vi "Setup array.vi"() -> (3 "output array":string[](array[string]))   [LabVIEW 2014]
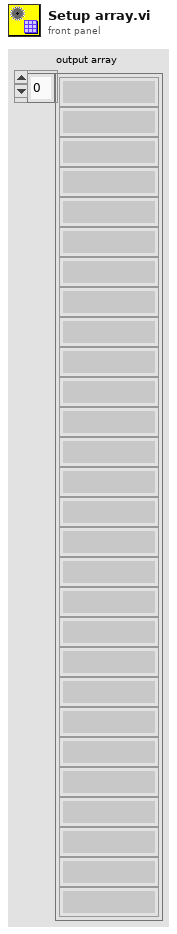
[diagram p1: front panel]
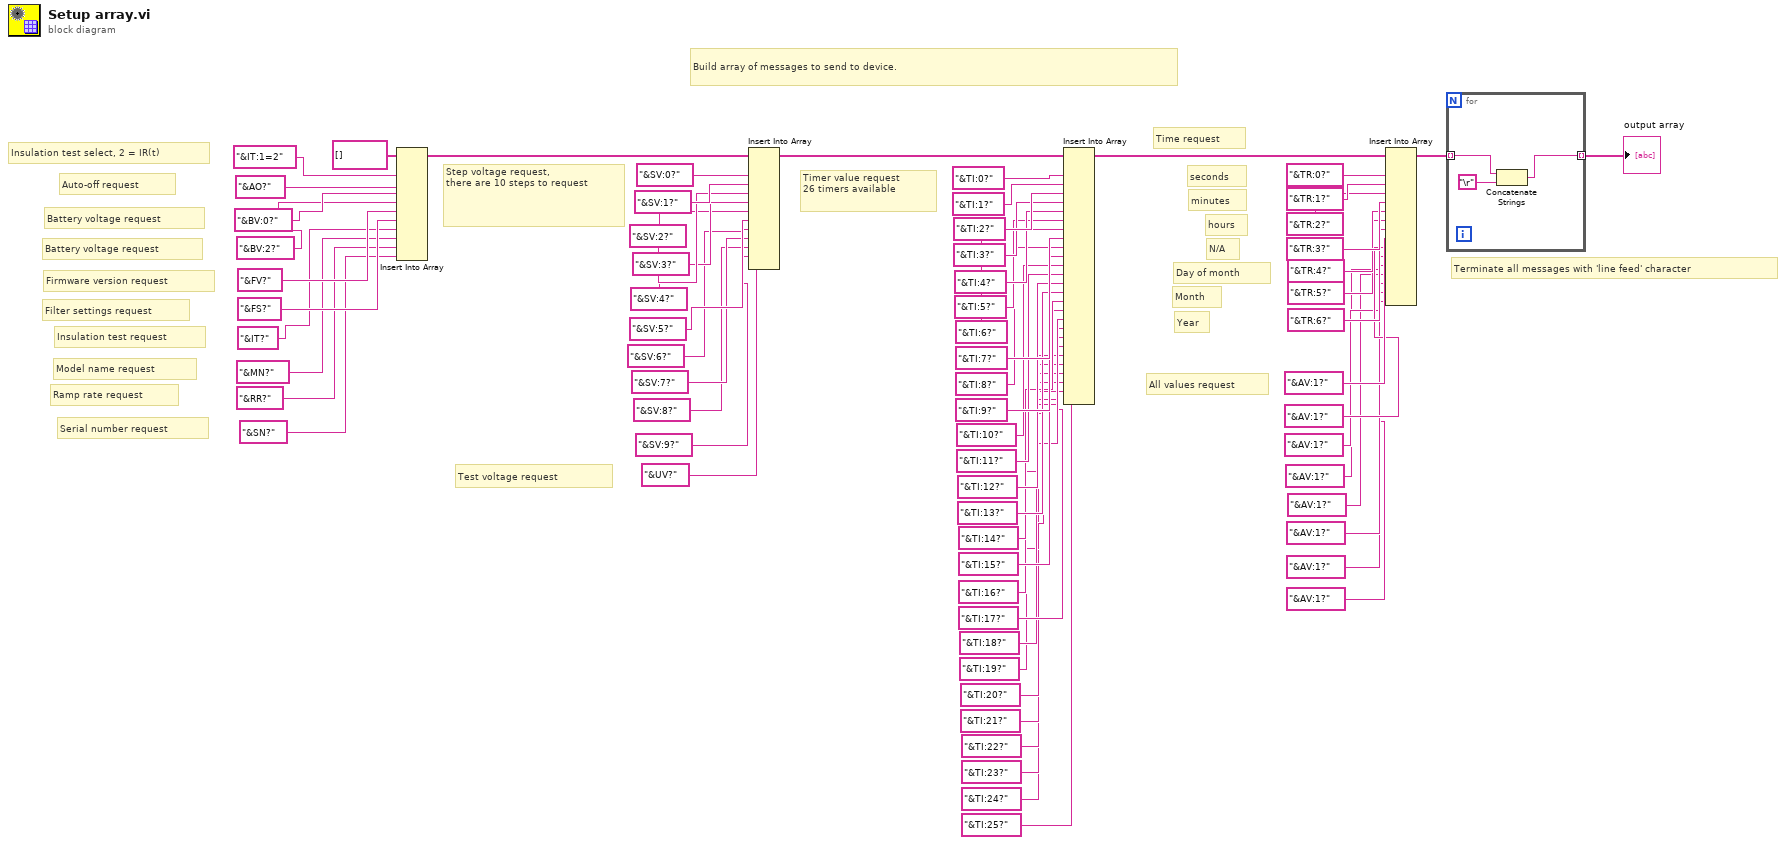
[diagram p0: block diagram]
diagram:
  # "Terminate all messages with 'line feed' character"
  # "All values request"
  # "Year"
  # "Month"
  # "Day of month"
  # "N/A"
  # "hours"
  # "minutes"
  # "seconds"
  # "Time request"
  # "Timer value request\n26 timers available"
  # "Test voltage request"
  # "Step voltage request,\nthere are 10 steps to request"
  # "Build array of messages to send to device."
  # "Serial number request"
  # "Ramp rate request"
  # "Model name request"
  # "Insulation test request"
  # "Filter settings request"
  # "Firmware version request"
  # "Battery voltage request"
  # "Battery voltage request"
  # "Auto-off request"
  # "Insulation test select, 2 = IR(t)"
  n1 = Insert Into Array(array=string[] [], new element #1="&IT:1=2", new element #2="&AO?", new element #3="&BV:0?", new element #4="&BV:2?", new element #5="&FV?", new element #6="&FS?", new element #7="&IT?", new element #8="&MN?", new element #9="&RR?", new element #10="&SN?") -> (w55:string[])  [unwired: 1 in]
  n2 = Insert Into Array(array=w55, new element #1="&SV:0?", new element #2="&SV:1?", new element #3="&SV:2?", new element #4="&SV:3?", new element #5="&SV:4?", new element #6="&SV:5?", new element #7="&SV:6?", new element #8="&SV:7?", new element #9="&SV:8?", new element #10="&SV:9?", new element #11="&UV?") -> (w19:string[])  [unwired: 1 in]
  n3 = Insert Into Array(array=w19, new element #1="&TI:0?", new element #2="&TI:1?", new element #3="&TI:2?", new element #4="&TI:3?", new element #5="&TI:4?", new element #6="&TI:5?", new element #7="&TI:6?", new element #8="&TI:7?", new element #9="&TI:8?", new element #10="&TI:9?", new element #11="&TI:10?", new element #12="&TI:11?", new element #13="&TI:12?", new element #14="&TI:13?", new element #15="&TI:14?", new element #16="&TI:15?", new element #17="&TI:16?", new element #18="&TI:17?", new element #19="&TI:18?", new element #20="&TI:19?", new element #21="&TI:20?", new element #22="&TI:21?", new element #23="&TI:22?", new element #24="&TI:23?", new element #25="&TI:24?", new element #26="&TI:25?") -> (w11:string[])  [unwired: 1 in]
  n4 = Insert Into Array(array=w11, new element #1="&TR:0?", new element #2="&TR:1?", new element #3="&TR:2?", new element #4="&TR:3?", new element #5="&TR:4?", new element #6="&TR:5?", new element #7="&TR:6?", new element #8="&AV:1?", new element #9="&AV:1?", new element #10="&AV:1?", new element #11="&AV:1?", new element #12="&AV:1?", new element #13="&AV:1?", new element #14="&AV:1?", new element #15="&AV:1?") -> (w10:string[])  [unwired: 1 in]
  n5 = for {
    tunnel: [w70] -> w67 mode=indexing
    tunnel: w10 -> [w71] mode=indexing
    n6 = Concatenate Strings(w71, "\r") -> (w70:string)
  }
  "output array" <- w67
